vi "Do.vi"(8 "error in (no error)":errorcluster, 10 "Actor in":refnum<class "Actor.lvclass">, 11 "Set Output Value Msg":refnum<class "Set Output Value Msg.lvclass">) -> (0 "error out":errorcluster, 2 "Actor out":refnum<class "Actor.lvclass">)   [LabVIEW 2017, in "BNT_DAQmx.lvlib" / "Set Output Value Msg.lvclass"]
doc: "This VI delivers the message to the actor by calling the appropriate method(s) on the actor."
uses:
  Set Output Value Msg.lvclass
  <vilib>/ActorFramework/Actor/Actor.lvclass
  C:/User/Brand/LVP/Detlab/GemDiscProduction/Packages/CSPP_Core/Messages/CSPP_PVUpdate Msg/CSPP_PVUpdate Msg.lvclass
  BNT_DAQmx-MCSV/BNT_DAQmx-MCSV.lvclass
  C:/Program Files (x86)/National Instruments/LabVIEW 2017/vi.lib/ActorFramework/Actor/Actor.lvclass
  BNT_DAQmx-MCSV/BNT_DAQmx-MCSV.lvclass/BNT_DAQmx-MCSV.ctl
  CSPP_Core/Messages/CSPP_PVUpdate Msg/CSPP_PVUpdate Msg.lvclass/CSPP_PVUpdate Msg.ctl
  CSPP_Core/Classes/CSPP_ProcessVariables/ProcessVariable/PV.lvclass/PV.ctl
  Set Output Value Msg.lvclass/Set Output Value Msg.ctl
  CSPP_Core/Classes/CSPP_ProcessVariables/ProcessVariable/PV.lvclass
  CSPP_Core/Messages/CSPP_PVUpdate Msg/CSPP_PVUpdate Msg.lvclass
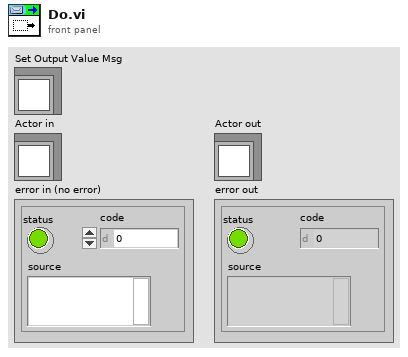
[diagram p1: front panel]
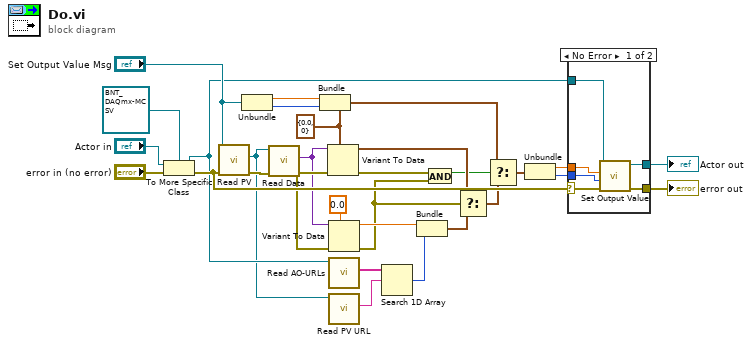
[diagram p0: block diagram]
diagram:
  w24 = cluster{"Value":dbl, "Channel":i32} {"Value"=0.0, "Channel"=0} ("Type")
  n1 = To More Specific Class(target class=refnum<class "BNT_DAQmx-MCSV.lvclass"> refnum ("Actor in"), reference="Actor in", error in="error in (no error)") -> (specific class reference=w10:refnum<class "BNT_DAQmx-MCSV.lvclass">, error out=w21:errorcluster)
  n2 = call "Read PV.vi"("error in (no error)"=w21, "CSPP_PVUpdate Msg in"="Set Output Value Msg") -> ("error out"=w26:errorcluster, "PV"=w2:refnum<class "PV.lvclass">)  [unwired: 7 in, 1 out]
  n3 = Unbundle ("Pre-Unbundler")("Set Output Value Msg") -> (w18:dbl, w17:i32)
  n4 = call "Read Data.vi"("error in (no error)"=w26, "PV in"=w2) -> ("error out"=w15:errorcluster, "Data"=w9:variant)  [unwired: 7 in, 1 out]
  n5 = Bundle ("Pre-Bundler")(cluster=w24, "Value"=w18, "Channel"=w17) -> (w25:cluster{"Value":dbl, "Channel":i32})
  n6 = Variant To Data(error in=w15, type=w24, Variant=w9) -> (data=w13:cluster{"Value":dbl, "Channel":i32}, error out=w14:errorcluster)
  n7 = Variant To Data(error in=w15, type=0.0 ("Value"), Variant=w9) -> (data=w7:dbl, error out=w3:errorcluster)
  n8 = call "Read AO-URLs.vi"("BNT_DAQmx-MCSV in"=w10) -> ("AO-URLs"=w8:string[])  [unwired: 9 in, 1 out]
  n9 = call "Read PV URL.vi"("PV in"=w2) -> ("PV URL"=w1:string)  [unwired: 8 in, 2 out]
  n10 = Search 1D Array(1D array=w8, element=w1) -> (index of element=w6:i32)  [unwired: 1 in]
  n11 = Bundle ("Pre-Bundler")("Value"=w7, "index of element"=w6) -> (w5:cluster{"Value":dbl, "index of element":i32})  [unwired: 1 in]
  n12 = And(x=w14, y=w3) -> (x .and. y?=w4:bool)
  n13 = Select ("MainSelect")(t=w13, s=w3, f=w5) -> (s? t:f=w12:cluster{"Value":dbl, "index of element":i32})
  n14 = Select ("MainSelect")(t=w25, s=w4, f=w12) -> (s? t:f=w23:cluster{"Value":dbl, "index of element":i32})
  n15 = Unbundle ("Main-Unbundler")(w23) -> ("Value"=w20:dbl, "index of element"=w19:i32)
  n16 = case shown="No Error" w21 {
    selector: w21 -> [w34 w38]
    tunnel: [w36 w38] -> w29
    tunnel: [w35 w37] -> w28
    tunnel: w10 -> [w31 w37]
    tunnel: w20 -> [w33 _]
    tunnel: w19 -> [w32 _]
    frame No Error {
      n17 = call "Set Output Value.vi"("Error In"=w34, "Channel"=w32, "Value"=w33, "BNT_DAQmx-MCSV in"=w31) -> ("Error Out"=w36:errorcluster, "BNT_DAQmx-MCSV out"=w35:refnum<class "BNT_DAQmx-MCSV.lvclass">)  [unwired: 6 in]
    }
    frame Error {
    }
  }
  "error out" <- w29
  "Actor out" <- w28
